vi "CANOpen_NMT Create Status Channels.vi"(7 "Channel":T2, 8 "error in (no error)":errorcluster, 9 "Parent Ref in":T1 format="%.0x", 11 "CANOpen Receive Status GUID":string) -> (0 "error out":errorcluster)   [LabVIEW 2021, in "CANOpen Addon System Explorer.lvlib"]
uses:
  CANOpen Addon System Explorer.lvlib
  <vilib>/NI VeriStand/Custom Device API/Custom Device Channel.ctl
  <vilib>/NI VeriStand/Custom Device API/Custom Device Channel Type.ctl
  <vilib>/NI VeriStand/Custom Device API/Custom Device Item Ref.ctl
  <vilib>/NI VeriStand/Custom Device API/Custom Device API.lvlib
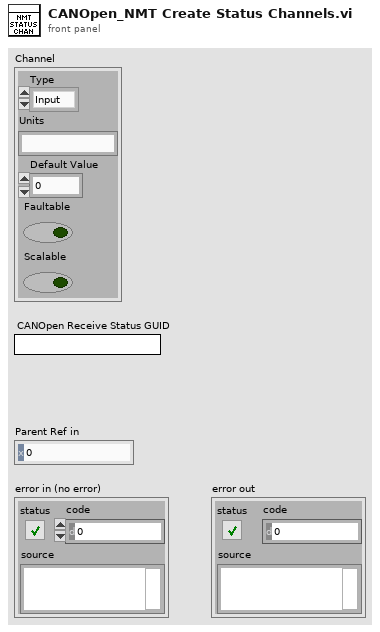
[diagram p1: front panel]
types:
  T1 = typedef "Custom Device API.lvlib/Custom Device Item Ref.ctl" = u64
  T2 = typedef "Custom Device API.lvlib/Custom Device Channel.ctl" = cluster{"Type":T3, "Units":string, "Default Value":dbl, "Faultable":bool, "Scalable":bool}
  T3 = typedef "Custom Device API.lvlib/Custom Device Channel Type.ctl" = enum16{"Input", "Output"}
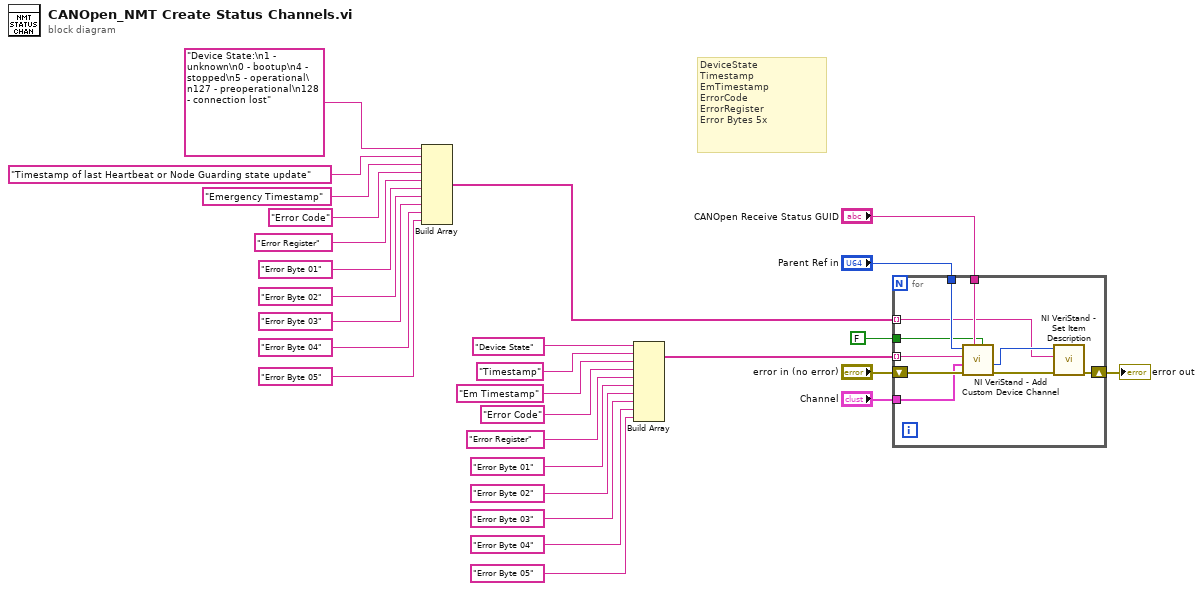
[diagram p0: block diagram]
diagram:
  # "DeviceState\nTimestamp\nEmTimestamp\nErrorCode\nErrorRegister\nError Bytes 5x"
  n1 = Build Array("Device State:\n1 - unknown\n0 - bootup\n4 - stopped\n5 - operational\n127 - preoperational\n128 - connection lost" ("CANOpen Receive Status GUID"), "Timestamp of last Heartbeat or Node Guarding state update" ("CANOpen Receive Status GUID"), "Emergency Timestamp" ("CANOpen Receive Status GUID"), "Error Code" ("CANOpen Receive Status GUID"), "Error Register" ("CANOpen Receive Status GUID"), "Error Byte 01" ("CANOpen Receive Status GUID"), "Error Byte 02" ("CANOpen Receive Status GUID"), "Error Byte 03" ("CANOpen Receive Status GUID"), "Error Byte 04" ("CANOpen Receive Status GUID"), "Error Byte 05" ("CANOpen Receive Status GUID")) -> (w2:string[])
  n2 = Build Array("Device State" ("CANOpen Receive Status GUID"), "Timestamp" ("CANOpen Receive Status GUID"), "Em Timestamp" ("CANOpen Receive Status GUID"), "Error Code" ("CANOpen Receive Status GUID"), "Error Register" ("CANOpen Receive Status GUID"), "Error Byte 01" ("CANOpen Receive Status GUID"), "Error Byte 02" ("CANOpen Receive Status GUID"), "Error Byte 03" ("CANOpen Receive Status GUID"), "Error Byte 04" ("CANOpen Receive Status GUID"), "Error Byte 05" ("CANOpen Receive Status GUID")) -> (w15:string[])
  n3 = for {
    tunnel: "Parent Ref in" -> [w37]
    shift-right: [w34] -> w26
    shift-left: "error in (no error)" -> [w38]
    tunnel: w15 -> [w33] mode=indexing
    tunnel: "Channel" -> [w32]
    tunnel: "CANOpen Receive Status GUID" -> [w31]
    tunnel: w2 -> [w30] mode=indexing
    tunnel: FALSE ("Highlight? (F)") -> [w29]
    n4 = call <vilib>:"NI VeriStand - Add Custom Device Channel.vi"("Highlight? (F)"=w29, "GUID (Default Channel)"=w31, "error in (no error)"=w38, "Channel"=w32, "Channel Name"=w33, "Parent Ref in"=w37) -> ("error out"=w36:errorcluster, "Channel Ref"=w35:T1)  [unwired: 2 in, 2 out]
    n5 = call <vilib>:"NI VeriStand - Set Item Description.vi"("error in (no error)"=w36, "Description"=w30, "Item Ref in"=w35) -> ("error out"=w34:errorcluster)  [unwired: 6 in, 2 out]
  }
  "error out" <- w26
